vi "File_test.vi"() -> ()   [LabVIEW 2018]
panel:
  out "file or folder exists?":bool
  out "filenames":string[](array[string])
  out "folder names":string[](array[string])
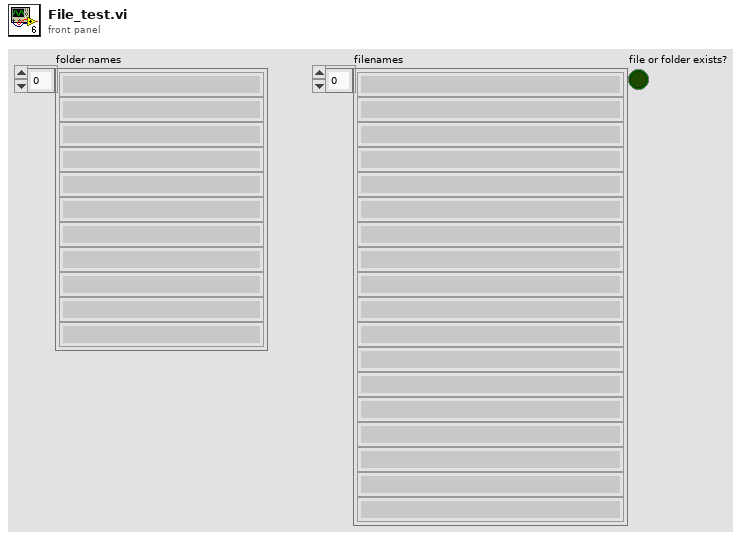
[diagram p1: front panel]
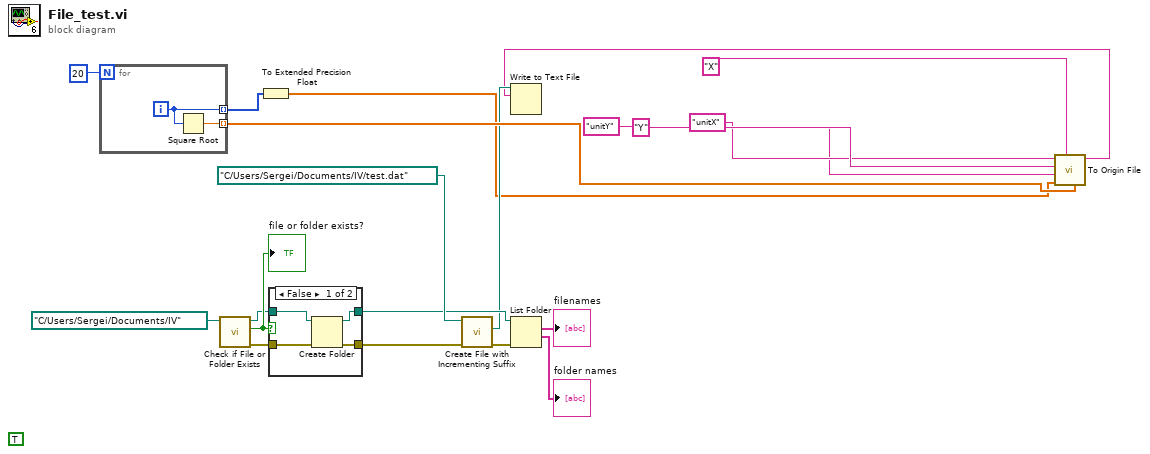
[diagram p0: block diagram]
diagram:
  (unwired) TRUE ("transpose? (no:F)")
  n1 = for {
    N: 20 -> [_]
    tunnel: [w22] -> w19 mode=indexing
    tunnel: [w21] -> w6 mode=indexing
    i -> [w21]
    n2 = Square Root(x=w21) -> (sqrt(x)=w22:dbl)
  }
  n3 = call <vilib>:"Check if File or Folder Exists.vi"("path"=path "C:/Users/Sergei/Documents/IV") -> ("error out"=w1:errorcluster, "file or folder exists?"=w3:bool, "dup path"=w2:path)  [unwired: 8 in]
  "file or folder exists?" <- w3
  n4 = To Extended Precision Float(1:w6) -> (0:w5:ext[])
  n5 = case shown="False" w3 {
    tunnel: w2 -> [w26 w27]
    tunnel: [w25 w28] -> w15
    tunnel: w1 -> [w24 w28]
    tunnel: [w23 w27] -> w14
    frame False {
      n6 = Create Folder(path (use dialog)=w26, error in=w24) -> (created path=w23:path, error out=w25:errorcluster)  [unwired: 1 in, 1 out]
    }
    frame True {
    }
  }
  n7 = call <vilib>:"Create File with Incrementing Suffix.vi"("error in (no error)"=w15, "file path"=path "C:/Users/Sergei/Documents/IV/test.dat") -> ("error out"=w13:errorcluster, "actual path"=w12:path)  [unwired: 7 in, 1 out]
  n8 = List Folder(path=w14, error in=w13) -> (filenames=→"filenames":string[], folder names=→"folder names":string[])  [unwired: 2 in, 2 out]
  n9 = call "To Origin File.vi"("Y"=w19, 7:"X" ("string"), "X"=w5, 9:"unitY" ("string"), 10:"Y" ("string"), "Prefix"="unitX" ("string")) -> ("Text"=w7:string)  [unwired: 5 in]
  n10 = Write to Text File(file (use dialog)=w12, text=w7) -> ()  [unwired: 2 in, 3 out]
